vi "teleop.vi"() -> ()   [LabVIEW 2010, in "LASA Beta.lvrbt"]
uses:
  LASA Beta.lvrbt
  <vilib>/NXT/Block Support/NXT_InputPort.ctl
  op-init.vi
  <vilib>/NXT/Dual Mode Library/Display/drawText.vi
  op-run.vi
  <vilib>/NXT/Dual Mode Library/Sensors/Touch_Pressed.vi
  <vilib>/NXT/Dual Mode Library/prims/inRangeAndCoerce/inRangeAndCoerce_float.vi
  <vilib>/NXT/Dual Mode Library/Display/drawNumber_float.vi
  <vilib>/NXT/Dual Mode Library/prims/inRangeAndCoerce/inRangeAndCoerce_int.vi
panel:
  in  "Manip Pos":dbl=127.0
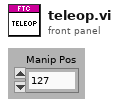
[diagram p1: front panel]
types:
  T1 = typedef "LVHSConnector.ctl" = cluster{"Hardware":string, "Flattened String":string}
  T2 = typedef "NXT_InputPort.ctl" = u8
  T3 = typedef "FTC ControllerState.ctl" = cluster{"Left X":i8, "Left Y":i8, "Right X":i8, "Right Y":i8, "Button Encoding 9-12":u8, "Button Encoding 1-8":u8, "POV":T4}
  T4 = typedef "FTC POVState.ctl" = i8
  T5 = typedef "FTC ButtonState.ctl" = cluster{"Button 1":bool, "Button 2":bool, "Button 3":bool, "Button 4":bool, "Button 5":bool, "Button 6":bool, "Button 7":bool, "Button 8":bool, "Button 9":bool, "Button 10":bool, "Button 11":bool, "Button 12":bool, "POV":T4}
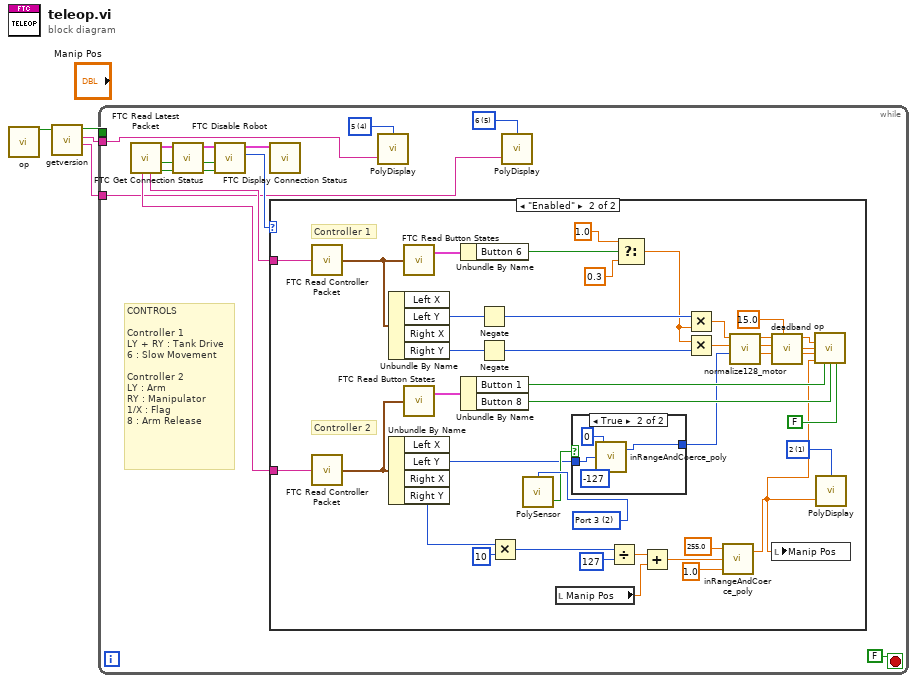
[diagram p0: block diagram]
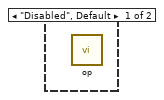
[diagram p2: hidden frame]
diagram:
  n1 = call-poly "op.vi"() -> ("Chain OUT"=w4:bool)  [unwired: 15 in]
  n2 = call "getversion.vi"("Chain IN"=w4) -> ("Revision"=w1:string, "Version"=w2:string, "Chain OUT"=w3:bool)  [unwired: 8 in]
  n3 = while {
    tunnel: w3 -> [_]
    tunnel: w2 -> [w6]
    tunnel: w1 -> [w5]
    stop <- FALSE stop-if-true
    w7 = i16 5 items=["1", "2", "3", "4", "5", "6", "7", "8"] ("Line")
    w8 = i16 4 items=["1", "2", "3", "4", "5", "6", "7", "8"] ("Line")
    # "CONTROLS\n\nController 1\nLY + RY : Tank Drive\n6 : Slow Movement\n\nController 2\nLY : Arm\nRY : Manipulator\n1/X : Flag\n8 : Arm Release"
    n4 = call <vilib>:"FTC Read Latest Packet.vi"() -> ("Packet Received?"=w19:bool, "Stopped?"=w17:bool, "NXT"=w18:T1, "Controller 1"=w14:string, "Controller 2"=w9:string)  [unwired: 6 in, 1 out]
    n5 = call <vilib>:"FTC Get Connection Status.vi"("Packet Received?"=w19, "Stopped?"=w17, "NXT"=w18) -> ("Online?"=w15:bool, "Stopped?"=w16:bool, "NXT"=w12:T1)  [unwired: 5 in]
    n6 = call <vilib>:"FTC Disable Robot.vi"("Online?"=w15, "Stopped?"=w16, "NXT"=w12) -> ("Enabled?"=w13:enum16{"Disabled", "Enabled"}, "NXT"=w11:T1)  [unwired: 3 in]
    n7 = call <vilib>:"FTC Display Connection Status.vi"("NXT"=w11) -> ()  [unwired: 10 in, 1 out]
    n8 = case shown="\"Enabled\"" w13 {
      tunnel: w14 -> [_ w60]
      tunnel: w9 -> [_ w59]
      frame "Disabled", Default {
        n9 = call-poly "op.vi"() -> ()  [unwired: 15 in, 1 out]
      }
      frame "Enabled" {
        w22 = i16 1 items=["1", "2", "3", "4", "5", "6", "7", "8"] ("Line")
        w27 = T2 2 items=["Port 1", "Port 2", "Port 3", "Port 4"] ("Port (Port 1)")
        # "Controller 2"
        # "Controller 1"
        n10 = call <vilib>:"FTC Read Controller Packet.vi"("Packet"=w60) -> ("Controller State"=w52:T3)  [unwired: 4 in]
        n11 = call <vilib>:"FTC Read Controller Packet.vi"("Packet"=w59) -> ("Controller State"=w58:T3)  [unwired: 4 in]
        n12 = Unbundle By Name(w52) -> ("Left Y"=w45:i8, "Right Y"=w54:i8)  [unwired: 2 out]
        n13 = Unbundle By Name(w58) -> ("Left Y"=w24:i8, "Right Y"=w44:i8)  [unwired: 2 out]
        n14 = call <vilib>:"FTC Read Button States.vi"("Controller State"=w52) -> ("Button States"=w51:T5)  [unwired: 2 in, 1 out]
        n15 = call <vilib>:"FTC Read Button States.vi"("Controller State"=w58) -> ("Button States"=w53:T5)  [unwired: 2 in, 1 out]
        n16 = Unbundle By Name(w51) -> ("Button 6"=w35:bool)
        n17 = Unbundle By Name(w53) -> ("Button 1"=w30:bool, "Button 8"=w29:bool)
        n18 = Negate(x=w45) -> (-x=w47:i8)
        n19 = Negate(x=w54) -> (-x=w46:i8)
        n20 = Multiply(x=w44, y=10) -> (x*y=w40:i32)
        n21 = call-poly <vilib>:"PolySensor.vi"("Port (Port 1)"=w27) -> ("Yes / No"=w26:bool)  [unwired: 2 in, 1 out]
        n22 = local read "Manip Pos"() -> (w42:dbl)
        n23 = case shown="True" w26 {
          tunnel: w24 -> [w61 w65]
          tunnel: [w61 w62] -> w25
          frame False {
          }
          frame True {
            n24 = call-poly <vilib>:"inRangeAndCoerce_poly.vi"("lower limit"=-127, "x"=w65, "upper limit"=0) -> ("coerced(x)"=w62:i32)  [unwired: 1 out]
          }
        }
        n25 = Divide(x=w40, y=127) -> (x/y=w39:dbl)
        n26 = Select(t=1.0 ("f"), s=w35, f=0.3) -> (s? t:f=w34:dbl)
        n27 = Add(x=w39, y=w42) -> (x+y=w38:dbl)
        n28 = Multiply(x=w47, y=w34) -> (x*y=w50:dbl)
        n29 = Multiply(x=w34, y=w46) -> (x*y=w49:dbl)
        n30 = call-poly <vilib>:"inRangeAndCoerce_poly.vi"("lower limit"=1.0, "x"=w38, "upper limit"=255.0) -> ("coerced(x)"=w23:dbl)  [unwired: 1 out]
        n31 = call "normalize128_motor.vi"("C"=w25, "B"=w49, "A"=w50) -> ("mC"=w55:dbl, "mB"=w56:dbl, "mA"=w57:dbl)  [unwired: 1 in, 1 out]
        n32 = call "deadband.vi"("Deadband"=15.0, "C"=w55, "B"=w56, "A"=w57) -> ("mC"=w31:dbl, "mB"=w32:dbl, "mA"=w33:dbl)  [unwired: 1 in, 1 out]
        n33 = local write "Manip Pos"(w23) -> ()
        n34 = call-poly "op.vi"("Left Drive"=w33, "Right Drive"=w32, "Arm"=w31, "Manipulator Position"=w23, "Flag"=w30, "Arm Release"=w29, "Auto Servo"=FALSE) -> ()  [unwired: 8 in, 1 out]
        n35 = call-poly <vilib>:"PolyDisplay.vi"("number"=w23, "Line"=w22) -> ()  [unwired: 2 in, 1 out]
      }
    }
    n36 = call-poly <vilib>:"PolyDisplay.vi"("Text"=w6, "Line"=w8) -> ()  [unwired: 2 in, 1 out]
    n37 = call-poly <vilib>:"PolyDisplay.vi"("Text"=w5, "Line"=w7) -> ()  [unwired: 2 in, 1 out]
  }
